vi "x1refTOx1refdot.vi"(10 "x1_ref_norm":dbl, 11 "Array: x1_ref_norm":dbl[](array[numeric])) -> (2 "Array: x1_ref_norm":dbl[](array[numeric]), 3 "x1_ref_norm_dot":dbl)   [LabVIEW 2013]
uses:
  <vilib>/Analysis/NI_AALPro.lvlib
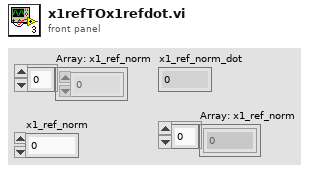
[diagram p1: front panel]
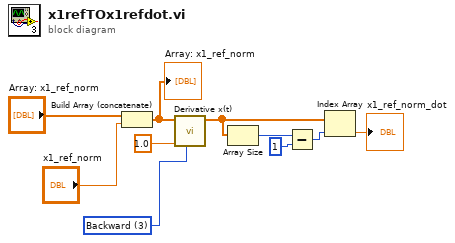
[diagram p0: block diagram]
diagram:
  w1 = u16 3 items=["2nd Order Central", "4th Order Central", "Forward", "Backward"] ("method")
  n1 = Build Array (concatenate)("Array: x1_ref_norm", "x1_ref_norm") -> (w7:dbl[])
  "Array: x1_ref_norm" <- w7
  n2 = call <vilib>:"Derivative x(t).vi"("method"=w1, "dt"=1.0, "X"=w7) -> ("dX/dt"=w6:dbl[])  [unwired: 7 in, 1 out]
  n3 = Array Size(array=w6) -> (size(s)=w5:i32)
  n4 = Subtract(x=w5, y=1) -> (x-y=w3:i32)
  n5 = Index Array(array=w6, index=w3) -> (element=→"x1_ref_norm_dot":dbl)
